vi "setting_yaw.vi"(9 "Numeric":sgl format="%#_13g", 11 "start":bool) -> (3 "yaw_speed":sgl, 10 "set_yaw":dbl)   [LabVIEW 2015]
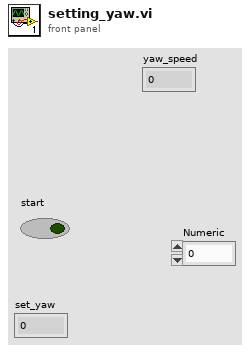
[diagram p1: front panel]
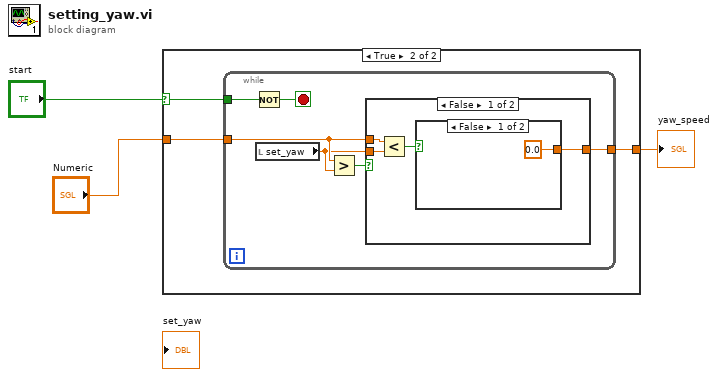
[diagram p0: block diagram]
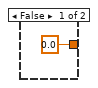
[diagram p2: hidden frame]
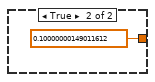
[diagram p3: hidden frame]
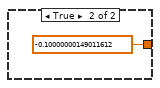
[diagram p4: hidden frame]
diagram:
  n1 = case shown="True" "start" {
    selector: "start" -> [_ w7]
    tunnel: "Numeric" -> [_ w6]
    tunnel: [sgl 0.0 w5] -> w1
    frame False {
    }
    frame True {
      n2 = while {
        tunnel: w7 -> [w13]
        tunnel: w6 -> [w9]
        tunnel: [w10] -> w5
        stop <- w12 stop-if-true
        n3 = Not(x=w13) -> (.not. x?=w12:bool)
        n4 = local read "set_yaw"() -> (w8:dbl)
        n5 = Greater?(x=w9, y=w8) -> (0:w11:bool)
        n6 = case shown="False" w11 {
          tunnel: [w14 sgl -0.1] -> w10
          tunnel: w9 -> [w17 _]
          tunnel: w8 -> [w16 _]
          frame False {
            n7 = Less?(x=w17, y=w16) -> (x < y?=w15:bool)
            n8 = case shown="False" w15 {
              tunnel: [sgl 0.0 sgl 0.1] -> w14
              frame False {
              }
              frame True {
              }
            }
          }
          frame True {
          }
        }
      }
    }
  }
  "yaw_speed" <- w1
